vi "digital data.vi"(8 "error in":errorcluster, 10 "Digital Signals":bool[](array[boolean])) -> (0 "error out":errorcluster)   [LabVIEW 2020, in "Acquisition .lvlib"]
doc: "acquire the digital data\n_____\nCreated using Delacor QMH Event Scripter 6.0.0.121."
uses:
  Acquisition .lvlib
  digital data Argument--cluster.ctl
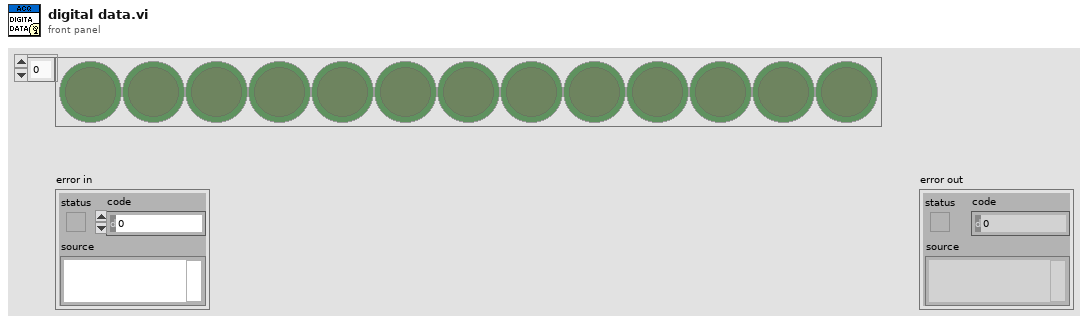
[diagram p1: front panel]
types:
  T1 = typedef "Acquisition .lvlib/digital data Argument--cluster.ctl" = cluster{"Digital Signals":bool[]}
  T2 = typedef "Acquisition .lvlib/Broadcast Events--cluster.ctl" = cluster{"Module Did Init":refnum<user-event>, "Status Updated":refnum<user-event>, "Error Reported":refnum<user-event>, "Module Did Stop":refnum<user-event>, "Update Module Execution Status":refnum<user-event>, "analog data":refnum<user-event>, "digital data":refnum<user-event>, "Digital Metdata has been acquired":refnum<user-event>}
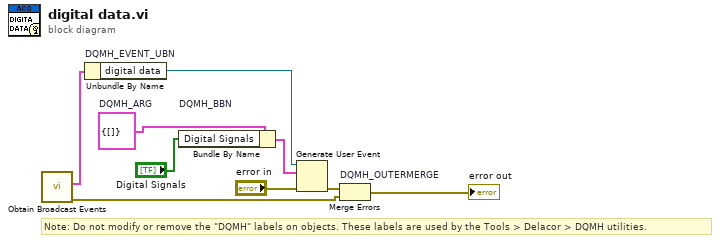
[diagram p0: block diagram]
diagram:
  w4 = T1 {"Digital Signals"=[]}  # DQMH_ARG
  # "Note: Do not modify or remove the \"DQMH\" labels on objects. These labels are used by the Tools > Delacor > DQMH utilities."
  n1 = call "Obtain Broadcast Events.vi"() -> ("error out"=w2:errorcluster, "Acquisition  Broadcast Events"=w1:T2)  [unwired: 10 in]
  n2 = Unbundle By Name "DQMH_EVENT_UBN"(w1) -> ("digital data"=w6:refnum<user-event>)
  n3 = Bundle By Name "DQMH_BBN"(cluster=w4, "Digital Signals"="Digital Signals") -> (w7:T1)
  n4 = Generate User Event(user event=w6, event data cluster=w7, error in="error in") -> (error out=w5:errorcluster)  [unwired: 1 in, 1 out]
  n5 = Merge Errors "DQMH_OUTERMERGE"(w5, w2) -> (→"error out":errorcluster)
